vi "Move Cell.vi"(8 "error in (no error)":errorcluster, 10 "Up/Down":bool=TRUE, 11 "Run Block in":refnum<class "Run Block.lvclass">) -> (0 "error out":errorcluster, 3 "Run Block out":refnum<class "Run Block.lvclass">)   [LabVIEW 2020, in "Run Utilities.lvlib" / "Run Block.lvclass"]
doc: "Move a cell up or down in the schedule based on the inner index selector. The selector can be specified via the <b>Select Cell.vi</b> (or Index selector property node)."
uses:
  Run Block.lvclass
  Run Block.lvclass/Run Block.ctl
  Schedule/Schedule.lvclass
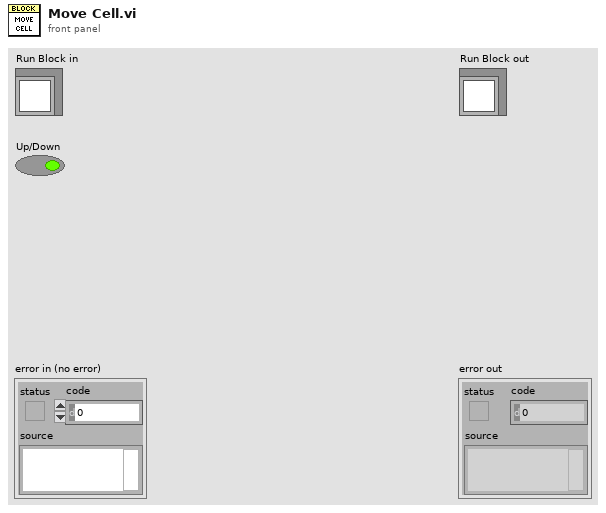
[diagram p1: front panel]
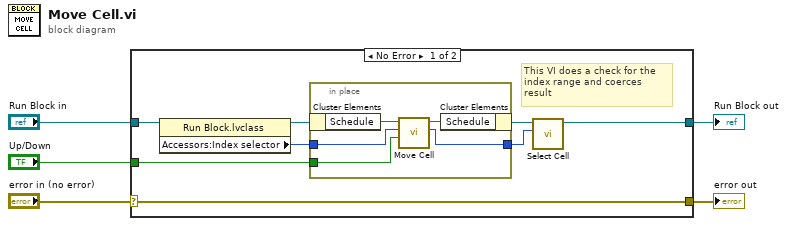
[diagram p0: block diagram]
diagram:
  n1 = case shown="No Error" "error in (no error)" {
    selector: "error in (no error)" -> [w13 w20]
    tunnel: [w13 w20] -> w4
    tunnel: [w7 w19] -> w2
    tunnel: "Run Block in" -> [w12 w19]
    tunnel: "Up/Down" -> [w11 _]
    frame No Error {
      # "This VI does a check for the index range and coerces result"
      n2 = property class="Run Block.lvclass"(reference=w12) -> (reference out=w10:refnum<class "Run Block.lvclass">, "Accessors:Index selector"=w9:i32)  [unwired: 1 in, 1 out]
      n3 = in-place {
        in-place-border: w11 -> [w16]
        in-place-border: w9 -> [w15]
        in-place-border: [w14] -> w6
        n4 = in-place-cluster #1(w10) -> ("Schedule"=w18:refnum<class "Schedule.lvclass">)
        n5 = call-dynamic "Move Cell.vi"("Up/Down"=w16, "Cell index"=w15, "Schedule in"=w18) -> ("New index"=w14:i32, "Schedule out"=w17:refnum<class "Schedule.lvclass">)  [unwired: 6 in, 1 out]
        n6 = in-place-cluster #1("Schedule"=w17) -> (w8:refnum<class "Run Block.lvclass">)
      }
      n7 = call-dynamic "Select Cell.vi"("Index selector"=w6, "Run Block in"=w8) -> ("Run Block out"=w7:refnum<class "Run Block.lvclass">)  [unwired: 8 in, 1 out]
    }
    frame Error {
    }
  }
  "error out" <- w4
  "Run Block out" <- w2
